vi "readCmdSetup.vi"(0 "refnum in":T2, 11 "error in (no error)":errorcluster) -> (4 "refnum out":T2, 6 "cmdSetup":T1={"DefaultQueueName"="", "responseTimeout"=10000, "logPostdata"="", "logResponse"=""}, 15 "error out":errorcluster)   [LabVIEW 2017]
uses:
  <vilib>/Utility/config.llb/Config Data RefNum.ctl
  cmdSetup.ctl
  <vilib>/Utility/config.llb/Read Key (String).vi
  <vilib>/Utility/config.llb/Read Key (I32).vi
  <vilib>/Utility/config.llb/NI_LVConfig.lvlib
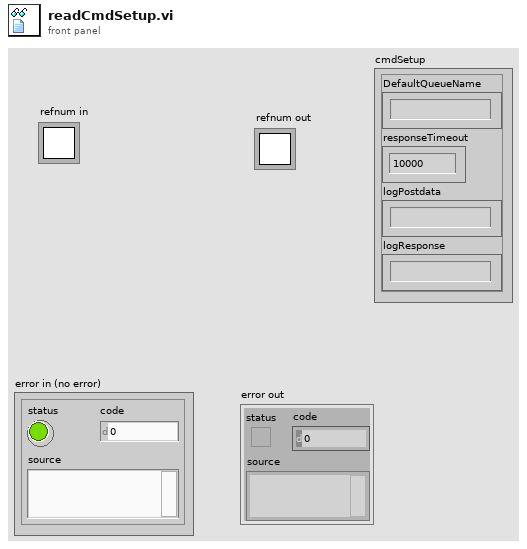
[diagram p1: front panel]
types:
  T1 = typedef "cmdSetup.ctl" = cluster{"DefaultQueueName":string, "responseTimeout":i32, "logPostdata":string, "logResponse":string}
  T2 = typedef "NI_LVConfig.lvlib/Config Data RefNum.ctl" = refnum<k1>
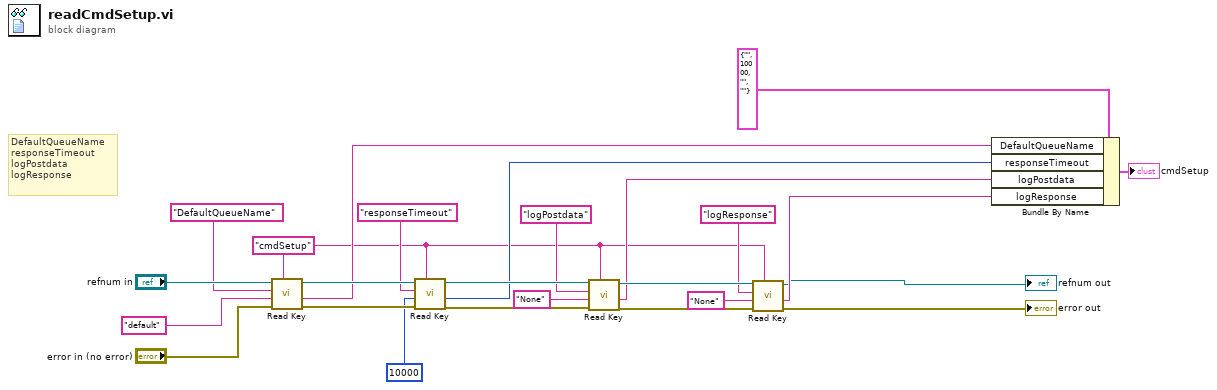
[diagram p0: block diagram]
diagram:
  w3 = "cmdSetup" ("section")
  # "DefaultQueueName\nresponseTimeout\nlogPostdata\nlogResponse"
  n1 = call-poly <vilib>:"Read Key.vi"("section"=w3, "error in (no error)"="error in (no error)", "default value"="default", "key"="DefaultQueueName", "refnum"="refnum in") -> ("error out"=w20:errorcluster, "value"=w8:string, "refnum out"=w21:T2)  [unwired: 3 in, 1 out]
  n2 = call-poly <vilib>:"Read Key.vi"("section"=w3, "error in (no error)"=w20, "default value"=10000, "key"="responseTimeout", "refnum"=w21) -> ("error out"=w16:errorcluster, "value"=w7:i32, "refnum out"=w17:T2)  [unwired: 3 in, 1 out]
  n3 = call-poly <vilib>:"Read Key.vi"("section"=w3, "error in (no error)"=w16, "default value"="None", "key"="logPostdata", "refnum"=w17) -> ("error out"=w12:errorcluster, "value"=w6:string, "refnum out"=w13:T2)  [unwired: 3 in, 1 out]
  n4 = call-poly <vilib>:"Read Key.vi"("section"=w3, "error in (no error)"=w12, "default value"="None", "key"="logResponse", "refnum"=w13) -> ("error out"=→"error out":errorcluster, "value"=w5:string, "refnum out"=→"refnum out":T2)  [unwired: 3 in, 1 out]
  n5 = Bundle By Name(cluster=T1 {"DefaultQueueName"="", "responseTimeout"=10000, "logPostdata"="", "logResponse"=""} ("cmdSetup"), "DefaultQueueName"=w8, "responseTimeout"=w7, "logPostdata"=w6, "logResponse"=w5) -> (→"cmdSetup":T1)
